vi "Evaluate Boolean Evaluation Trigger (Array).vi"(8 "error in (no error)":errorcluster, 10 "Trigger Data":dbl[](array[numeric]), 11 "Boolean Evaluation Trigger in":refnum<class "Boolean Evaluation Trigger.lvclass">) -> (0 "error out":errorcluster, 1 "Trigger indices":i32[](array[numeric]), 2 "Trigger":bool, 3 "Boolean Evaluation Trigger out":refnum<class "Boolean Evaluation Trigger.lvclass">)   [LabVIEW 2015, in "Boolean Evaluation Trigger.lvclass"]
uses:
  Boolean Evaluation Trigger.lvclass
  Boolean Evaluation Trigger.lvclass/Boolean Evaluation Trigger.ctl
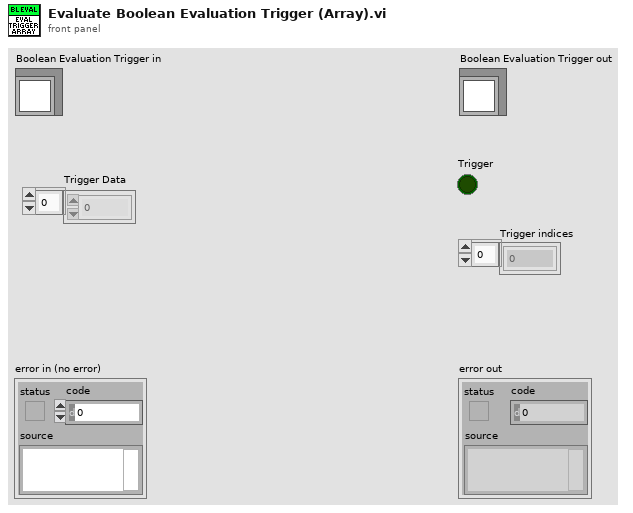
[diagram p1: front panel]
types:
  T1 = typedef "Boolean Evaluation Trigger.lvclass/Operand.ctl" = enum16{"==", "!=", "<", "<=", ">", ">="}
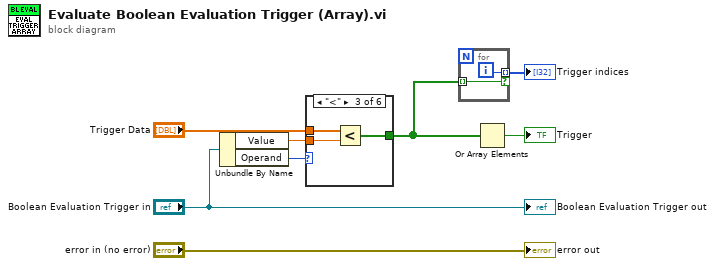
[diagram p0: block diagram]
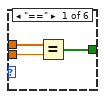
[diagram p2: hidden frame]
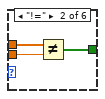
[diagram p3: hidden frame]
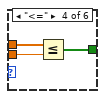
[diagram p4: hidden frame]
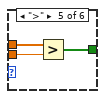
[diagram p5: hidden frame]
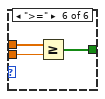
[diagram p6: hidden frame]
diagram:
  n1 = Unbundle By Name("Boolean Evaluation Trigger in") -> ("Value"=w4:dbl, "Operand"=w8:T1)
  n2 = case shown="\"<\"" w8 {
    tunnel: "Trigger Data" -> [w10 w13 w16 w19 w22 w25]
    tunnel: w4 -> [w11 w14 w17 w20 w23 w26]
    tunnel: [w9 w12 w15 w18 w21 w24] -> w2
    frame "==" {
      n3 = Equal?(x=w10, y=w11) -> (x = y?=w9:bool[])
    }
    frame "!=" {
      n4 = Not Equal?(x=w13, y=w14) -> (x != y?=w12:bool[])
    }
    frame "<" {
      n5 = Less?(x=w16, y=w17) -> (x < y?=w15:bool[])
    }
    frame "<=" {
      n6 = Less Or Equal?(x=w19, y=w20) -> (x <= y?=w18:bool[])
    }
    frame ">" {
      n7 = Greater?(x=w22, y=w23) -> (0:w21:bool[])
    }
    frame ">=" {
      n8 = Greater Or Equal?(x=w25, y=w26) -> (x >= y?=w24:bool[])
    }
  }
  n9 = for {
    tunnel: w2 -> [w27] mode=indexing
    tunnel: [w28] -> w1 mode=indexing if=w27
    i -> [w28]
  }
  "Trigger indices" <- w1
  n10 = Or Array Elements(Boolean array=w2) -> (logical OR=→"Trigger":bool)
  "error out" <- "error in (no error)"
  "Boolean Evaluation Trigger out" <- "Boolean Evaluation Trigger in"
